vi "Update Move Up-Down Button Enabled State.vi"(11 "UI Data in":refnum<class "Settings UI.lvclass">) -> (3 "UI Data out":refnum<class "Settings UI.lvclass">)   [LabVIEW 2020, in "Output Sequencer.lvlib" / "Settings UI.lvclass"]
uses:
  Settings UI.lvclass
  Settings UI.lvclass/Settings UI.ctl
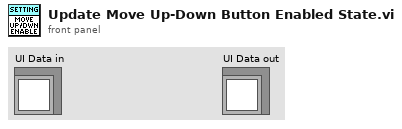
[diagram p1: front panel]
types:
  T1 = enum8{"Enabled", "Disabled", "Disabled and Grayed Out"}
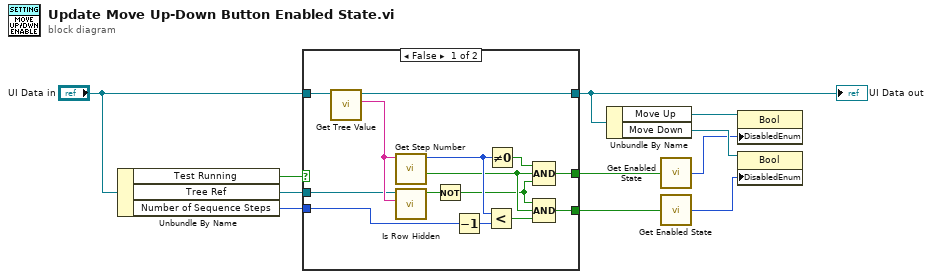
[diagram p0: block diagram]
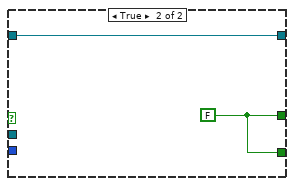
[diagram p2: hidden frame]
diagram:
  n1 = Unbundle By Name("UI Data in") -> ("Test Running"=w1:bool, "Tree Ref"=w4:refnum<vi>, "Number of Sequence Steps"=w3:i32)
  n2 = case shown="False" w1 {
    tunnel: "UI Data in" -> [w25 w27]
    tunnel: [w19 w26] -> w8
    tunnel: [w18 w26] -> w6
    tunnel: w4 -> [w16 _]
    tunnel: w3 -> [w13 _]
    tunnel: [w12 w27] -> w2
    frame False {
      n3 = call "Get Tree Value.vi"("UI Data in"=w25) -> ("Value"=w17:string, "UI Data out"=w12:refnum<class "Settings UI.lvclass">)  [unwired: 9 in]
      n4 = call "Get Step Number.vi"("Tree Tag"=w17) -> ("Is Step tag?"=w20:bool, "Step Number"=w22:i32)  [unwired: 8 in, 1 out]
      n5 = call "Is Row Hidden.vi"("Tag"=w17, "TreeControl in"=w16) -> ("Hidden"=w15:bool)  [unwired: 9 in]
      n6 = Not(x=w15) -> (.not. x?=w14:bool)
      n7 = Decrement(x=w13) -> (x-1=w23:i32)
      n8 = Less?(x=w22, y=w23) -> (x < y?=w21:bool)
      n9 = Not Equal To 0?(x=w22) -> (x != 0?=w24:bool)
      n10 = Compound Arithmetic op=AND(w24, w20, w14) -> (w19:bool)
      n11 = Compound Arithmetic op=AND(w14, w20, w21) -> (w18:bool)
    }
    frame True {
      w26 = FALSE
    }
  }
  "UI Data out" <- w2
  n12 = Unbundle By Name(w2) -> ("Move Up"=w9:refnum<vi>, "Move Down"=w10:refnum<vi>)
  n13 = call "Get Enabled State.vi"("Enabled?"=w8) -> ("State"=w7:T1)
  n14 = call "Get Enabled State.vi"("Enabled?"=w6) -> ("State"=w5:T1)
  n15 = property on="Property Node" class="Bool"(reference=w9, "DisabledEnum"=w7) -> ()  [unwired: 1 in, 2 out]
  n16 = property on="Property Node" class="Bool"(reference=w10, "DisabledEnum"=w5) -> ()  [unwired: 1 in, 2 out]
